vi "solar Create.vi"(5 "Default LVClass":refnum<class "solar.lvclass">, 7 "AddonVIs":refnum<vi>[](array[refnum]), 8 "error in (no error)":errorcluster, 9 "VI Refnum":refnum<vi>, 10 "VI MenuRef":refnum<k9>, 11 "Target":string) -> (0 "error out":errorcluster, 1 "Is Main?":bool, 2 "UserEvent":refnum<user-event>, 3 "solar":refnum<class "solar.lvclass">)   [LabVIEW 2018, in "solar.lvclass"]
doc: "This creates and initializes a SOLAR target by name. If this is the top level main target, this loads the application settings from the solar.ini configuration file, launches the SOLAR user interface, initializes the SOLAR addons and launches the splash screen. Each target loads its LabVIEW Class from the target's configuration file. Specify the Default LVClass to load."
uses:
  solar.lvclass
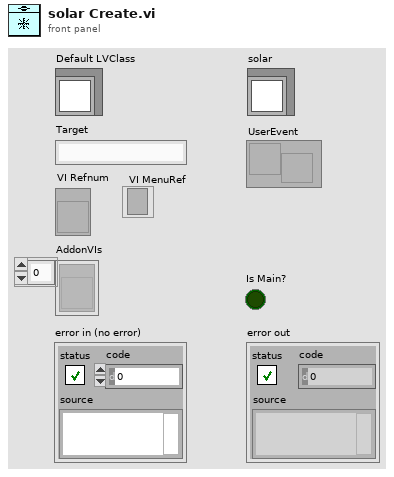
[diagram p1: front panel]
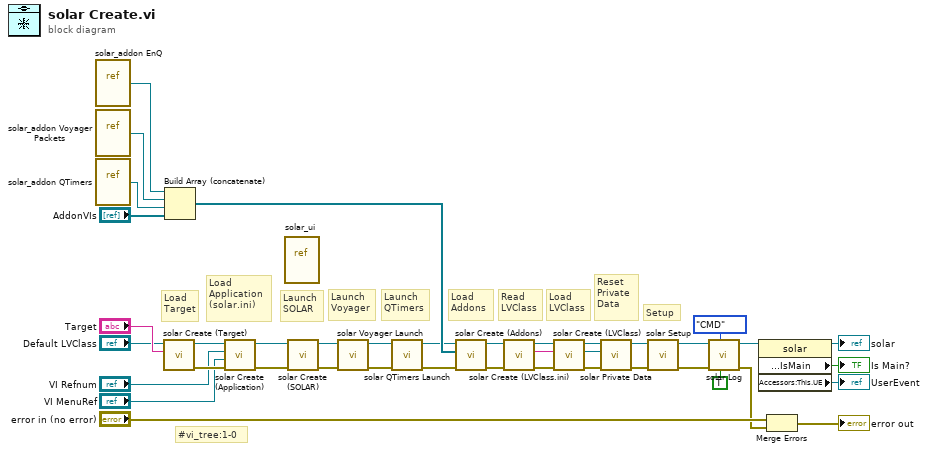
[diagram p0: block diagram]
diagram:
  # "Launch\nQTimers"
  # "#vi_tree:1-0"
  # "Launch\nVoyager"
  # "Launch\nSOLAR"
  # "Setup"
  # "Reset\nPrivate\nData"
  # "Load\nLVClass"
  # "Read\nLVClass"
  # "Load\nAddons"
  # "Load\nApplication\n(solar.ini)"
  # "Load\nTarget"
  n1 = vi-ref "solar_addon EnQ.vi"() -> (w34:refnum<vi>)
  n2 = vi-ref "solar_addon Voyager Packets.vi"() -> (w7:refnum<vi>)
  n3 = vi-ref "solar_addon QTimers.vi"() -> (w6:refnum<vi>)
  n4 = call "solar Create (Target).vi"("Target Name"="Target", "Default LVClass"="Default LVClass") -> ("error out"=w29:errorcluster, "solar"=w30:refnum<class "solar.lvclass">)  [unwired: 8 in]
  n5 = Build Array (concatenate)(w34, w7, w6, "AddonVIs") -> (w27:refnum<vi>[])
  n6 = call "solar Create (Application).vi"("error in (no error)"=w29, "Menu"="VI MenuRef", "VI"="VI Refnum", "Default LVClass"=w30) -> ("error out"=w13:errorcluster, "solar out"=w12:refnum<class "solar.lvclass">)  [unwired: 6 in]
  n7 = vi-ref "solar_ui.vi"() -> ()  [unwired: 1 out]
  n8 = call "solar Create (SOLAR).vi"("error in (no error)"=w13, "solar in"=w12) -> ("error out"=w11:errorcluster, "solar out"=w10:refnum<class "solar.lvclass">)  [unwired: 8 in]
  n9 = call "solar Voyager Launch.vi"("error in (no error)"=w11, "solar in"=w10) -> ("error out"=w5:errorcluster, "solar out"=w3:refnum<class "solar.lvclass">)  [unwired: 8 in]
  n10 = call "solar QTimers Launch.vi"("error in (no error)"=w5, "solar in"=w3) -> ("error out"=w4:errorcluster, "solar out"=w2:refnum<class "solar.lvclass">)  [unwired: 8 in]
  n11 = call "solar Create (Addons).vi"("error in (no error)"=w4, "AddonVIs"=w27, "Default LVClass"=w2) -> ("error out"=w19:errorcluster, "solar out"=w20:refnum<class "solar.lvclass">)  [unwired: 7 in]
  n12 = call "solar Create (LVClass.ini).vi"("error in (no error)"=w19, "Default LVClass"=w20) -> ("error out"=w22:errorcluster, "LVClass"=w21:string, "solar out"=w23:refnum<class "solar.lvclass">)  [unwired: 7 in]
  n13 = call "solar Create (LVClass).vi"("error in (no error)"=w22, "LVClass (*.lvclass)"=w21, "Default LVClass"=w23) -> ("error out"=w18:errorcluster, "dup Default LVClass"=w14:refnum<class "solar.lvclass">, "solar out"=w16:refnum<class "solar.lvclass">)  [unwired: 6 in]
  n14 = call-dynamic "solar Private Data.vi"("error in (no error)"=w18, "Default LVClass"=w14, "solar in"=w16) -> ("error out"=w17:errorcluster, "solar out"=w15:refnum<class "solar.lvclass">)  [unwired: 7 in]
  n15 = call-dynamic "solar Setup.vi"("error in (no error)"=w17, "solar in"=w15) -> ("error out"=w9:errorcluster, "solar out"=w8:refnum<class "solar.lvclass">)  [unwired: 8 in]
  n16 = call "solar Log.vi"("Clear Error? (T)"=TRUE ("Clear Error?"), "Type (TLM)"=enum8{"CMD", "TLM"}."CMD" ("Type (CMD)"), "error in (no error)"=w9, "solar in"=w8) -> ("error out"=w37:errorcluster, "solar out"=w39:refnum<class "solar.lvclass">)  [unwired: 6 in]
  n17 = property class="solar"(reference=w39) -> (reference out=→"solar":refnum<class "solar.lvclass">, "Accessors:Main.IsMain"=→"Is Main?":bool, "Accessors:This.UE"=→"UserEvent":refnum<user-event>)  [unwired: 1 in, 1 out]
  n18 = Merge Errors("error in (no error)", w37) -> (→"error out":errorcluster)
